vi "PI Discrete Controller.vi"() -> ()   [LabVIEW 2020]
uses:
  <vilib>/MakerHub/LINX/Public/Peripherals/Analog/Analog Read 1 Chan.vi
  <vilib>/MakerHub/LINX/Private/Local IO/LinxI2cWrite.vi
  <vilib>/MakerHub/LINX/Public/Utilities/Check Channel.vi
  <vilib>/MakerHub/LINX/Public/Peripherals/Analog/Analog Read N Chans.vi
  <vilib>/MakerHub/LINX/Private/Local IO/LinxAnalogRead.vi
  <vilib>/MakerHub/LINX/Public/Utilities/Open Serial.vi
  <vilib>/MakerHub/LINX/Private/Utilties/Generate Error.vi
  <vilib>/MakerHub/LINX/LMH-LINX.lvlib
panel:
  out "Salida":dynamicdata(graph)
  out "Señal de control":dbl(graph)
  out "r":dbl
  out "T":dbl
  out "IT":i32
  in  "SET":bool
  in  "Ref":dbl(slide) min=0.0 max=5.0 step=0.5 scale=0.0..5.0
  out "Error":dbl(graph)
  in  "tsim":dbl
  # "U(z)\n----\nE(z)"
  # "0.01656 + 0.01656 z^-1\n  ----------------------\n        2 - 2 z^-1"
  # "2.121 z^2 - 1.756 z + 0.04926\n  -----------------------------\n    2 z^2 - 2.814 z + 0.8137"
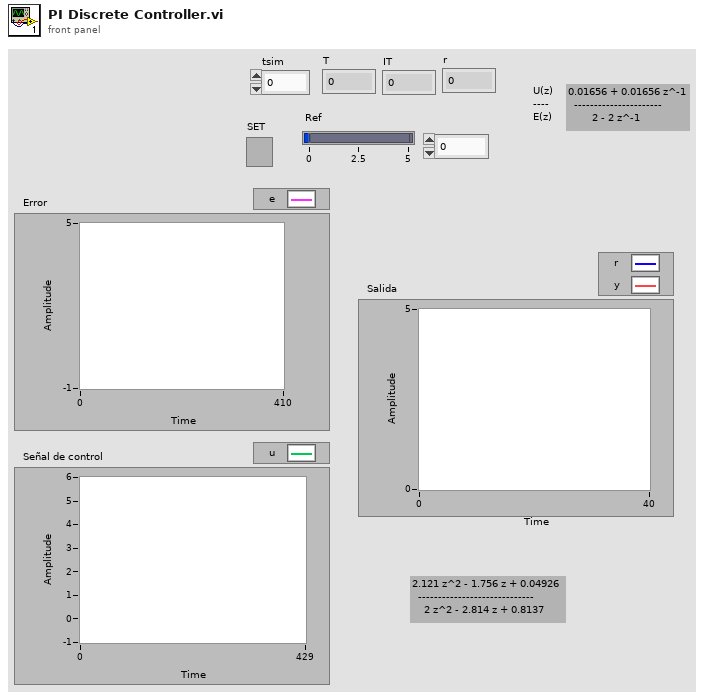
[diagram p1: front panel]
types:
  T1 = typedef "LMH-LINX.lvlib/LINX Ref.ctl" = cluster{"IO":T2, "Interface":T3, "LINX Device Config":T4}
  T2 = typedef "LMH-LINX.lvlib/Platform.ctl" = enum16{"Remote", "Local"}
  T3 = typedef "LMH-LINX.lvlib/Interface.ctl" = enum16{"Serial", "TCP"}
  T4 = typedef "LMH-LINX.lvlib/Device.lvlib/LINX Device Config.ctl" = cluster{"Interface":T3, "COM Port":refnum<visa-resource-name>, "TCP Configuration":T5, "Device Family":u8, "Device ID":u8, "Device Name":string, "TCP Ref":refnum<k5>, "Channels":T6}
  T5 = typedef "LMH-LINX.lvlib/Device.lvlib/TCP Config.ctl" = cluster{"IP Address":string, "Port":u16}
  T6 = typedef "LMH-LINX.lvlib/Channels.ctl" = cluster{"DI":u8[], "DO":u8[], "AI":u8[], "AO":u8[], "PWM":u8[], "QE":u8[], "UART":u8[], "I2C 2":u8[], "SPI":u8[], "CAN":u8[], "Servo":u8[], "AI Ref (V)":dbl, "AI Resolution (Bits)":u8, "AO Ref (V)":dbl, "AO Resolution (Bits)":u8}
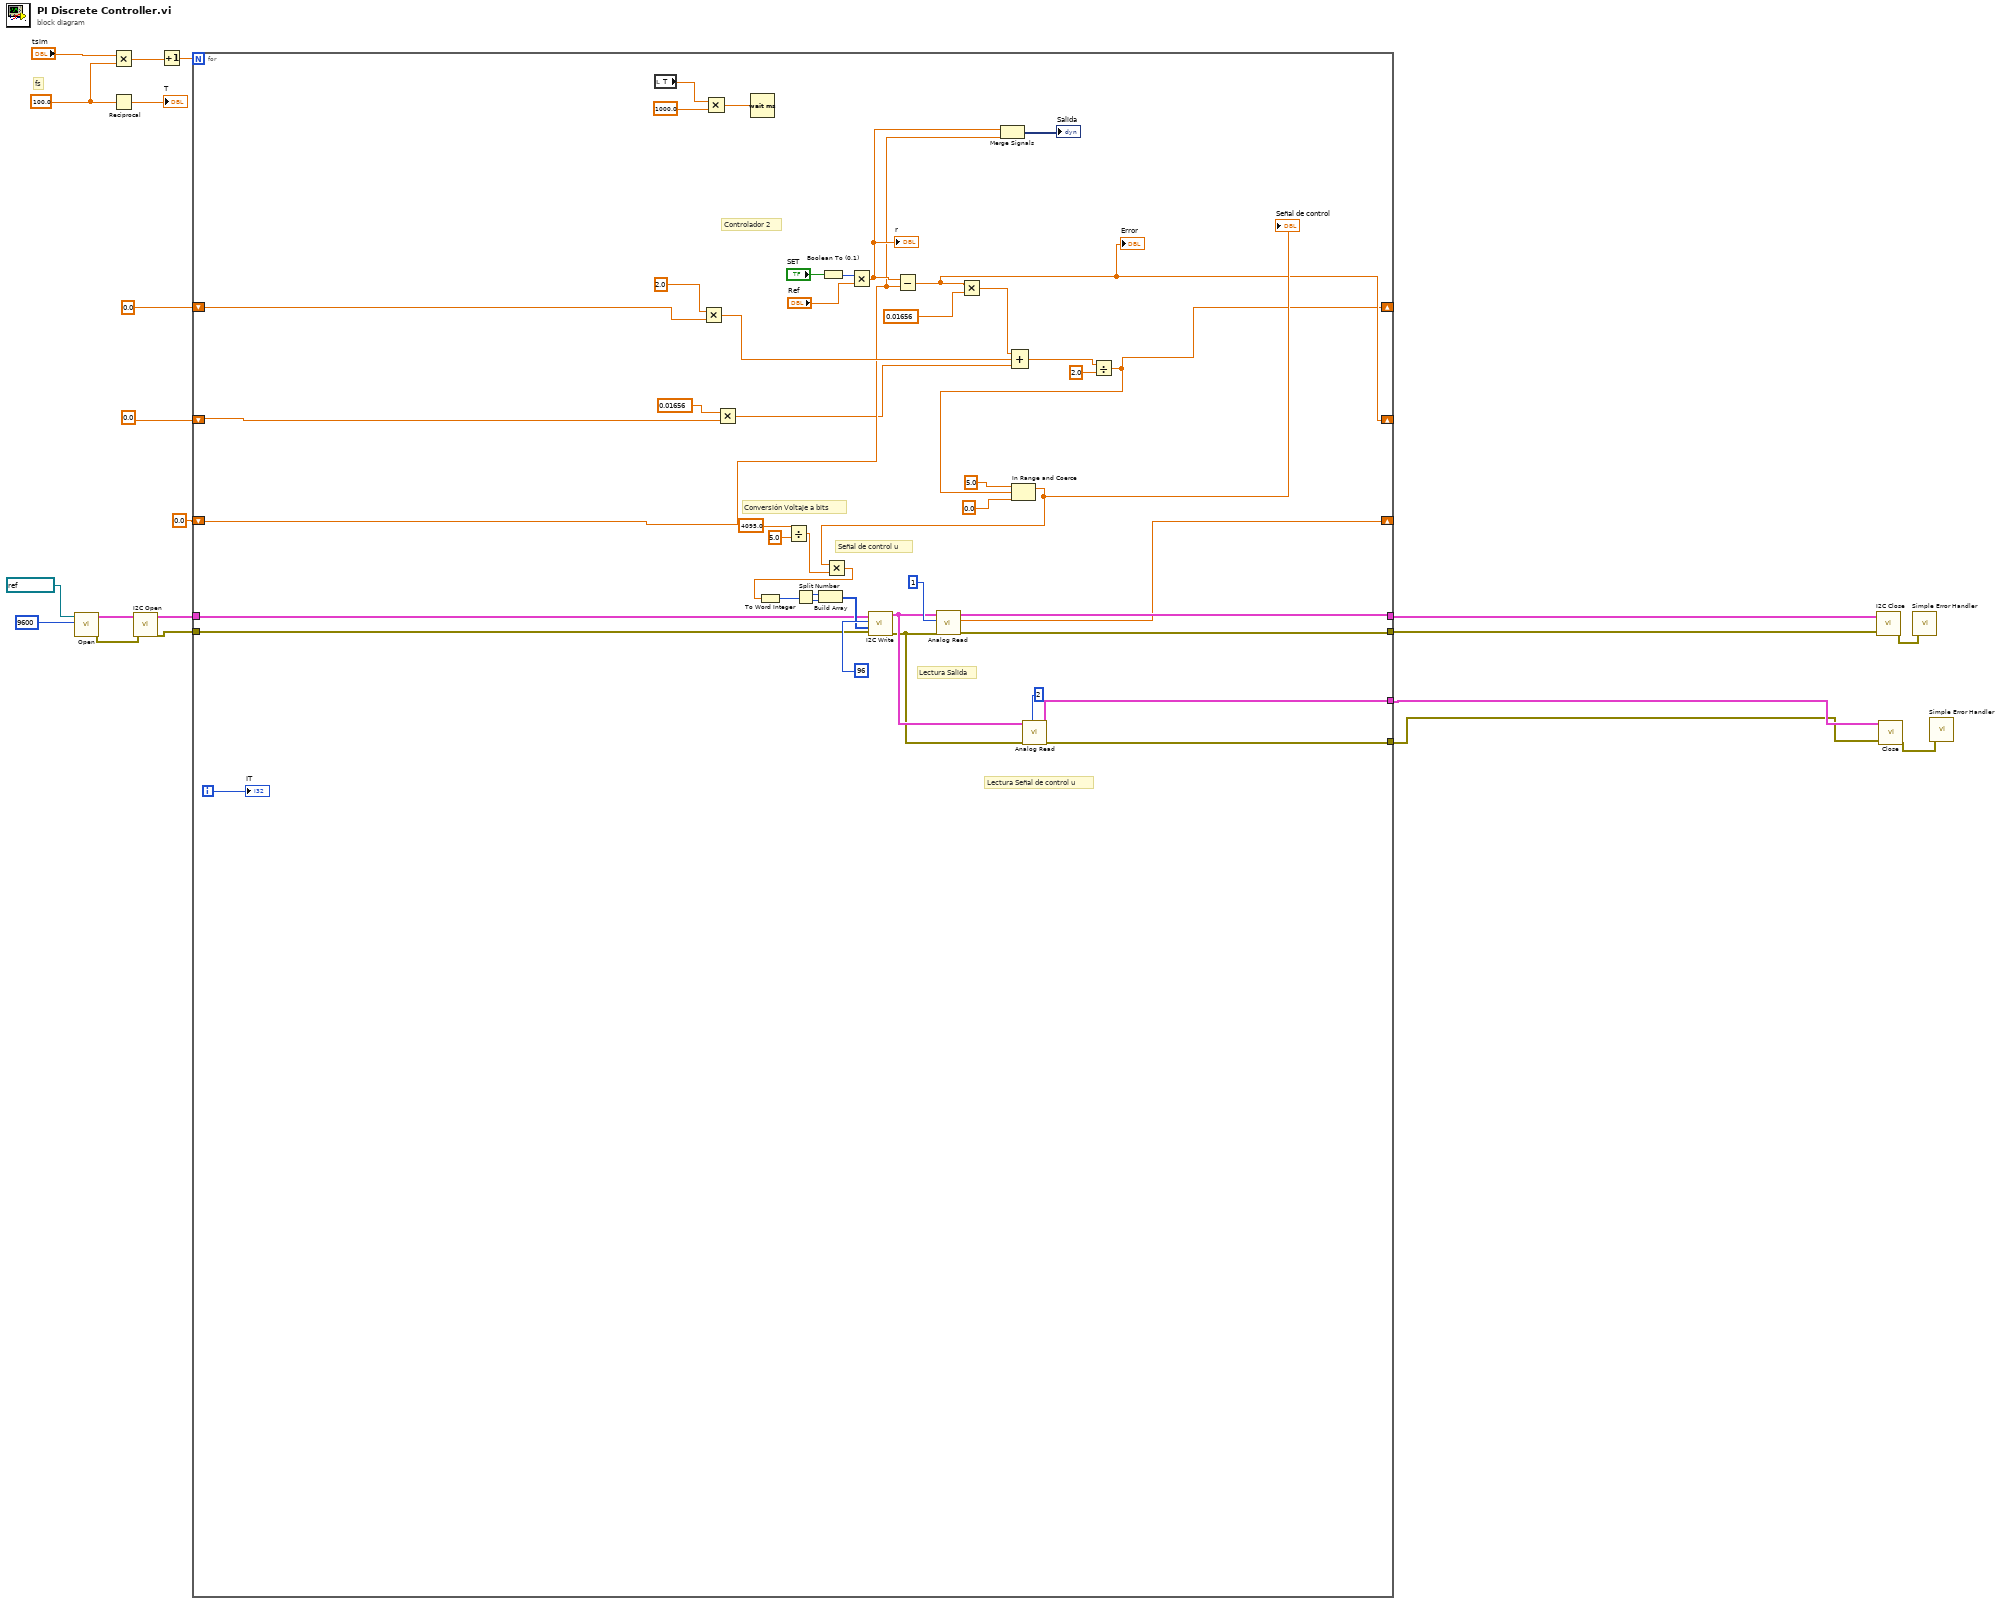
[diagram p0: block diagram]
diagram:
  w17 = 100.0 ("y")
  # "fs"
  n1 = call-poly <vilib>:"Open.vi"("Baud Rate Override"=u32 9600, "Serial Port"=refnum<visa-resource-name> "COM5") -> ("Error Out"=w12:errorcluster, "LINX Resource"=w13:T1)  [unwired: 7 in, 1 out]
  n2 = Multiply(x="tsim", y=w17) -> (x*y=w20:dbl)
  n3 = Reciprocal(x=w17) -> (1/x=→"T":dbl)
  n4 = call <vilib>:"I2C Open.vi"("Error In"=w12, "LINX Resource"=w13) -> ("Error Out"=w3:errorcluster, "LINX Resource"=w4:T1)  [unwired: 8 in]
  n5 = Increment(x=w20) -> (x+1=w19:dbl)
  n6 = for {
    N: w19 -> [_]
    shift-right: [w22] -> _
    shift-left: 0.0 -> [w30]
    shift-right: [w24] -> _
    shift-left: 0.0 -> [w35]
    shift-right: [w34] -> _
    shift-left: 0.0 ("Voltage") -> [w33]
    tunnel: w4 -> [w32]
    tunnel: [w39] -> w10
    tunnel: w3 -> [w31]
    tunnel: [w38] -> w9
    tunnel: [w26] -> w2
    tunnel: [w25] -> w1
    i -> [w62]
    # "Conversión Voltaje a bits"
    # "Señal de control u"
    # "Lectura Señal de control u"
    # "Lectura Salida"
    # "Controlador 2"
    n7 = local read "T"() -> (w65:dbl)
    n8 = Multiply(x=2.0, y=w30) -> (x*y=w55:dbl)
    n9 = Multiply(x=w65, y=1000.0) -> (x*y=w63:dbl)
    n10 = Multiply(x=0.01656, y=w35) -> (x*y=w21:dbl)
    n11 = Wait (ms)(milliseconds to wait=w63) -> ()  [unwired: 1 out]
    n12 = Divide ("Divide 2")(x=4095.0 ("Constant"), y=5.0 ("y 2")) -> (x/y=w45:dbl)
    n13 = Boolean To (0,1)(Boolean="SET") -> (0, 1=w60:i16)
    n14 = Multiply(x=w60, y="Ref") -> (x*y=w37:dbl)
    "r" <- w37
    n15 = Subtract(x=w37, y=w33) -> (x-y=w24:dbl)
    "Error" <- w24
    n16 = Multiply(x=w24, y=0.01656) -> (x*y=w23:dbl)
    n17 = Merge Signals(w37, w33) -> (→"Salida":dynamicdata)
    n18 = Compound Arithmetic op=ADD(w23, w55, w21) -> (w54:dbl)
    n19 = Divide(x=w54, y=2.0) -> (x/y=w22:dbl)
    n20 = In Range and Coerce(upper limit=5.0, x=w22, lower limit=0.0) -> (coerced(x)=w27:dbl)  [unwired: 1 out]
    "Señal de control" <- w27
    n21 = Multiply(x=w27, y=w45) -> (x*y=w44:dbl)
    n22 = To Word Integer(number=w44) -> (16bit integer=w48:i16)
    n23 = Split Number(x=w48) -> (hi(x)=w47:u8, lo(x)=w46:u8)
    n24 = Build Array ("Build Array 4")(w47, w46) -> (w43:u8[])
    n25 = call <vilib>:"I2C Write.vi"("Error In"=w31, "Data"=w43, "I2C Slave Address (0)"=u8 96, "LINX Resource"=w32) -> ("Error Out"=w40:errorcluster, "LINX Resource"=w41:T1)  [unwired: 6 in]
    n26 = call-poly <vilib>:"Analog Read.vi"("Error In"=w40, "Analog Channel"=u8 1 ("AO Channel"), "LINX Resource"=w41) -> ("Error Out"=w38:errorcluster, "Voltage"=w34:dbl, "LINX Resource"=w39:T1)  [unwired: 5 in, 1 out]
    n27 = call-poly <vilib>:"Analog Read.vi"("Error In"=w40, "Analog Channel"=u8 2, "LINX Resource"=w41) -> ("Error Out"=w25:errorcluster, "LINX Resource"=w26:T1)  [unwired: 5 in, 2 out]
    "IT" <- w62
  }
  n28 = call <vilib>:"I2C Close.vi"("Error In"=w9, "LINX Resource"=w10) -> ("Error Out"=w11:errorcluster)  [unwired: 8 in, 1 out]
  n29 = call <vilib>:"Close.vi"("Error In"=w1, "LINX Resource"=w2) -> ("Error Out"=w8:errorcluster)  [unwired: 9 in]
  n30 = call <vilib>:"Simple Error Handler.vi"("error in (no error)"=w11) -> ()  [unwired: 4 in, 5 out]
  n31 = call <vilib>:"Simple Error Handler.vi"("error in (no error)"=w8) -> ()  [unwired: 4 in, 5 out]
